vi "Calculate Waveform.vi"(8 "error in (no error)":errorcluster, 9 "Points":i16[](array[numeric]), 10 "Acquisition Time":timestamp, 11 "OWON SDS1022 in":refnum<class "SDS1000 Base CFG.lvclass">) -> (0 "error out":errorcluster, 2 "Waveform Graph":waveform(dbl)(graph), 3 "OWON SDS1022 out":refnum<class "SDS1000 Base CFG.lvclass">)   [LabVIEW 2023, in "OWON SDS1022.lvlib" / "SDS1000 Base CFG.lvclass"]
uses:
  Configurations/SDS1000 Base CFG/SDS1000 Base CFG.lvclass
  Configurations/SDS1000 Base CFG/SDS1000 Base CFG.lvclass/SDS1000 Base CFG.ctl
  5ff70b4c-a951-438e-aa90-247ca6a210be.vi
  b003ad20-f1c5-4d81-8556-46127c723614.vi
  <vilib>/JDP Science/JSONtext/Find Item.vi
  <vilib>/JDP Science/JSONtext/Next JSON Value.vi
  <vilib>/JDP Science/JSONtext/String Subset.vi
  <vilib>/JDP Science/JSONtext/Parsing/Advance past next JSON Value (inlined COPY).vi
  <vilib>/JDP Science/JSONtext/Parsing/Advance past whitespace.vi
  <vilib>/JDP Science/JSONtext/Parsing/Advance past String.vi
  <vilib>/JDP Science/JSONtext/Parsing/Advance past Number.vi
  <vilib>/JDP Science/JSONtext/Parsing/Advance past Line Ending.vi
  <vilib>/JDP Science/JSONtext/Parsing/Parse Full Path or Item Name.vi
  <vilib>/JDP Science/JSONtext/Parsing/Advance past Array.vi
  <vilib>/JDP Science/JSONtext/Parsing/Advance past Object.vi
  <vilib>/JDP Science/JSONtext/support/Error Cluster From Code.vi
  <vilib>/JDP Science/JSONtext/Offset/Find Item Locations by Path.vi
  <vilib>/JDP Science/JSONtext/JSON text to Variant.vi
  <vilib>/Utility/error.llb/Error Cluster From Error Code.vi
  <vilib>/JDP Science/JSONtext/LVClass Serializer/JSONtext LVClass Serializer.lvclass
  <vilib>/ErrorRing/Error Ring.xnode
  HAL/Configuration Base/Configuration Base.lvclass
panel:
  in  "Channel":u8(ring) items=["Channel 1"=1, "Channel 2"=2]
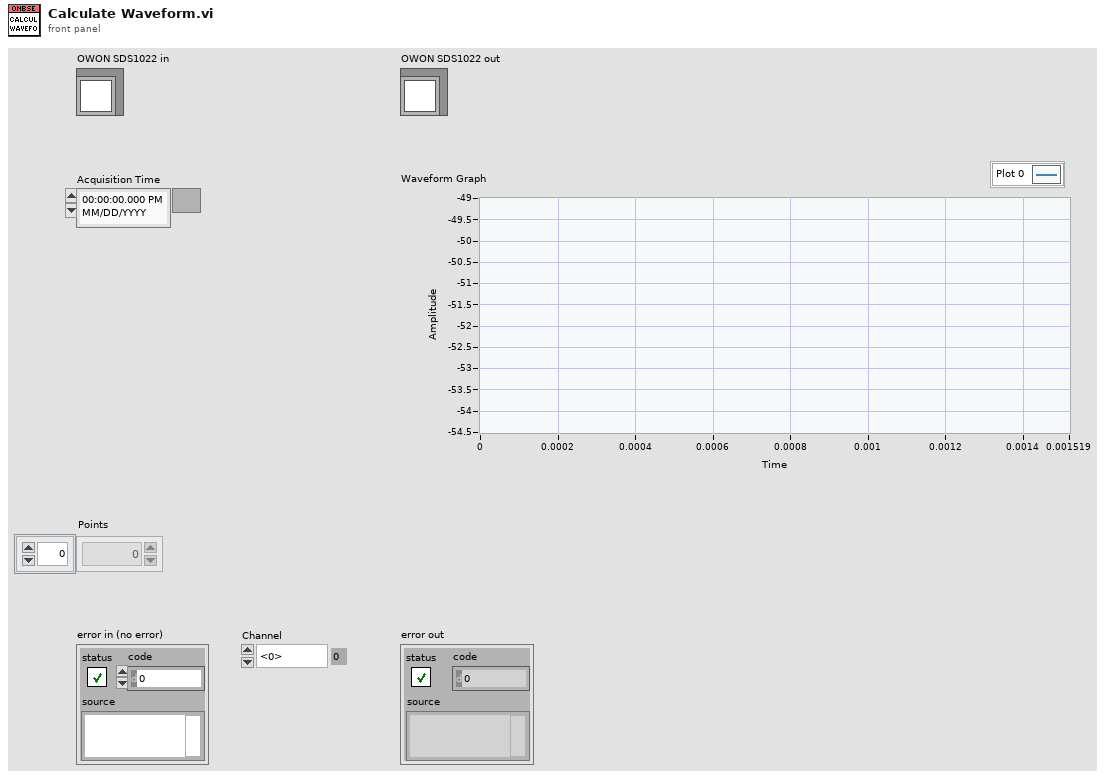
[diagram p1: front panel]
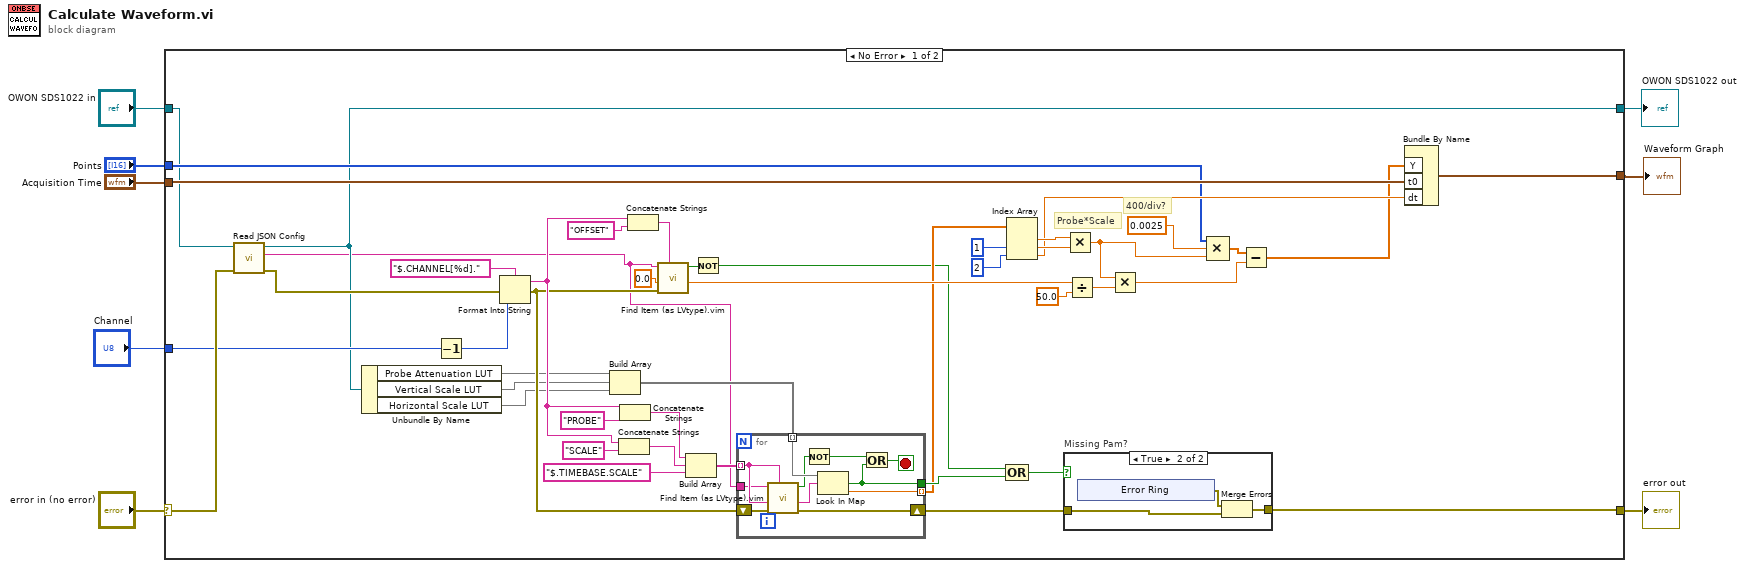
[diagram p0: block diagram]
diagram:
  n1 = case shown="No Error" "error in (no error)" {
    selector: "error in (no error)" -> [w54 w76]
    tunnel: [w52 w76] -> w7
    tunnel: [w10 w75] -> w5
    tunnel: "OWON SDS1022 in" -> [w11 w75]
    tunnel: "Points" -> [w13 _]
    tunnel: "Acquisition Time" -> [w51 _]
    tunnel: [w22 _] -> w2
    tunnel: "Channel" -> [w21 _]
    frame No Error {
      # "Probe*Scale"
      # "400/div?"
      n2 = call "Read JSON Config.vi"("error in (no error)"=w54, "object in"=w11) -> ("error out"=w12:errorcluster, "<JSON>Config"=w9:string, "object out"=w10:refnum<class "SDS1000 Base CFG.lvclass">)  [unwired: 7 in]
      n3 = Unbundle By Name(w10) -> ("Probe Attenuation LUT"=w35:map{string, dbl}, "Vertical Scale LUT"=w34:map{string, dbl}, "Horizontal Scale LUT"=w33:map{string, dbl})
      n4 = Decrement(x=w21) -> (x-1=w40:u8)
      n5 = Format Into String(format string="$.CHANNEL[%d].", error in=w12, w40) -> (resulting string=w45:string, error out=w43:errorcluster)  [unwired: 1 in]
      n6 = Build Array(w35, w34, w33) -> (w32:map{string, dbl}[])
      n7 = Concatenate Strings(w45, "SCALE" ("$Path or Item Name")) -> (w37:string)
      n8 = Concatenate Strings(w45, "PROBE" ("$Path or Item Name")) -> (w36:string)
      n9 = Concatenate Strings(w45, "OFFSET" ("$Path or Item Name")) -> (w48:string)
      n10 = call "Find Item (as LVtype).vim"("$Path or Item Name"=w48, "error in (no error)"=w43, "Data Type and Default Value"=0.0, "JSON"=w9) -> ("Data"=w42:dbl, "Found"=w24:bool)  [unwired: 4 in, 2 out]
      n11 = Build Array(w36, w37, "$.TIMEBASE.SCALE" ("$Path or Item Name")) -> (w38:string[])
      n12 = Not(x=w24) -> (.not. x?=w23:bool)
      n13 = for {
        tunnel: [w63] -> w30 mode=indexing
        tunnel: w38 -> [w62] mode=indexing
        tunnel: w9 -> [w60]
        shift-right: [w64] -> w53
        shift-left: w43 -> [w61]
        tunnel: w32 -> [w59] mode=indexing
        tunnel: [w55] -> w31
        stop <- w56 stop-if-true
        n14 = call "Find Item (as LVtype).vim"("$Path or Item Name"=w62, "error in (no error)"=w61, "Data Type and Default Value"=w62, "JSON"=w60) -> ("error out"=w64:errorcluster, "Data"=w65:string, "Found"=w58:bool)  [unwired: 4 in, 1 out]
        n15 = Not(x=w58) -> (.not. x?=w57:bool)
        n16 = Look In Map(map=w59, key=w65) -> (key not found?=w55:bool, value=w63:dbl)  [unwired: 1 in]
        n17 = Or(x=w57, y=w55) -> (x .or. y?=w56:bool)
      }
      n18 = Compound Arithmetic op=OR(w23, w31) -> (w50:bool)
      n19 = Index Array(array=w30, index #2=1 ("index"), index #3=2 ("index")) -> (element #1=w29:dbl, element #2=w27:dbl, element #3=w25:dbl)  [unwired: 1 in]
      n20 = case "Missing Pam?" shown="True" w50 {
        tunnel: w53 -> [w66 w68]
        tunnel: [w66 w67] -> w52
        frame False {
        }
        frame True {
          n21 = xnode "Error Ring"() -> ("error out"=w69:errorcluster)
          n22 = Merge Errors(w69, w68) -> (w67:errorcluster)
        }
      }
      n23 = Multiply(x=w29, y=w27) -> (x*y=w16:dbl)
      n24 = Divide(x=w42, y=50.0) -> (x/y=w17:dbl)
      n25 = Multiply(x=w16, y=w17) -> (x*y=w15:dbl)
      n26 = Compound Arithmetic op=MULTIPLY(w13, 0.0025, w16) -> (w20:dbl[])
      n27 = Subtract(x=w20, y=w15) -> (x-y=w14:dbl[])
      n28 = Bundle By Name("Y"=w14, "t0"=w51, "dt"=w25) -> (w22:waveform(dbl))  [unwired: 1 in]
    }
    frame Error {
    }
  }
  "error out" <- w7
  "OWON SDS1022 out" <- w5
  "Waveform Graph" <- w2
